vi "Init Sv.vi"   [LabVIEW 2019]
uses:
  TypeDef/SensorCalibrationData_Array.ctl
  TypeDef/SensorCalibrationData.ctl
  TypeDef/CalbrationPoint.ctl
  TypeDef/GUI Alarm customer settings.ctl
  TypeDef/GUI Alarm developer settings.ctl
  TypeDef/GUI Setting Channel.ctl
  TypeDef/Needle Valve Settings.ctl
  modbus engine custom/MB_ENGINE_class/Settings.ctl
  TypeDef/Channel Setting Array.ctl
  modbus engine custom/MB_ENGINE_class/MB_ENGINE.lvclass
types:
  T1 = typedef "Needle Valve Settings.ctl" = cluster{"average size":i32, "open force":u16, "close force":u16, "open settings":T2, "close settings":T2}
  T2 = typedef "MB_ENGINE.lvclass/Settings.ctl" = cluster{"ACC Steps Per Sec^2":u16, "DEC Steps Per Sec^2":u16, "Min Velosity Step Per Sec":u16, "Max Velosity Step Per Sec":u16, "MicroStep":u16}
  T3 = typedef "GUI Setting Channel.ctl" = cluster{"Name":string, "SensorID":u32}
  T4 = typedef "GUI Alarm developer settings.ctl" = cluster{"HIHI AI2":dbl, "HI AI2":dbl, "HIHI AI0":dbl, "HI AI0":dbl, "LOLO AI0":dbl, "LO AI0":dbl, "ENG2 OFF TIMEOUT":dbl, "ENG2 ON TIMEOUT":dbl, "HIHI AI3":dbl, "HI AI3":dbl, "HIHI AI1":dbl, "HI AI1":dbl, "LOLO AI1":dbl, "LO AI1":dbl, "ENG1 OFF TIMEOUT":dbl, "ENG1 ON TIMEOUT":dbl, "ENG0 OFF TIMEOUT":dbl, "ENG0 ON TIMEOUT":dbl, "LOLO AI8":dbl, "LO AI8":dbl, "LOLO AI9":dbl, "LO AI9":dbl, "LOLO AI5":dbl, "LO AI5":dbl, "Out Of Range HI":dbl, "Out Of Range LO":dbl}
  T5 = typedef "GUI Alarm customer settings.ctl" = cluster{"HIHI AI2":dbl, "HI AI2":dbl, "HIHI AI3":dbl, "HI AI3":dbl, "ENG0 OFF TIMEOUT":dbl, "ENG0 ON TIMEOUT":dbl, "HIHI AI7":dbl, "HI AI7":dbl, "HIHI AI6":dbl, "HI AI6":dbl, "HIHI AI5":dbl, "HI AI5":dbl}
  T6 = typedef "SensorCalibrationData_Array.ctl" = cluster{"SENSORS_ARR":T7[]}
  T7 = typedef "SensorCalibrationData.ctl" = cluster{"Name":string, "ID":u32, "Slope":dbl, "Intercept":dbl, "Calibration":T8[]}
  T8 = typedef "CalbrationPoint.ctl" = cluster{"RAW":dbl, "SCL":dbl}
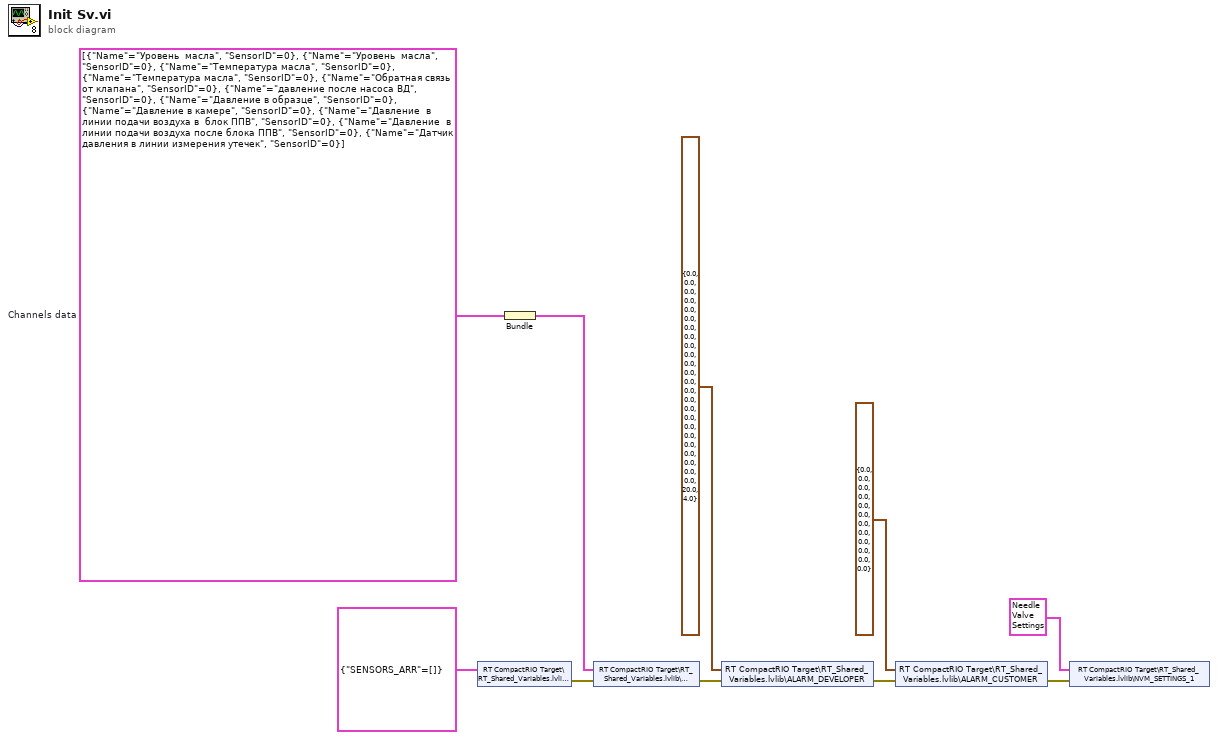
[diagram p0: block diagram]
diagram:
  w4 = T3[] [{"Name"="Уровень  масла", "SensorID"=0}, {"Name"="Уровень  масла", "SensorID"=0}, {"Name"="Температура масла", "SensorID"=0}, {"Name"="Температура масла", "SensorID"=0}, {"Name"="Обратная связь от клапана", "SensorID"=0}, {"Name"="давление после насоса ВД", "SensorID"=0}, {"Name"="Давление в образце", "SensorID"=0}, {"Name"="Давление в камере", "SensorID"=0}, {"Name"="Давление  в  линии подачи воздуха в  блок ППВ", "SensorID"=0}, {"Name"="Давление  в  линии подачи воздуха после блока ППВ", "SensorID"=0}, {"Name"="Датчик давления в линии измерения утечек", "SensorID"=0}]  # Channels data
  n1 = shared-variable "RT CompactRIO Target\\RT_Shared_Variables.lvlib\\SENSORS"(T6 {"SENSORS_ARR"=[]} ("SENSORS")) -> (error out=w9:errorcluster)  [unwired: 1 in]
  n2 = Bundle("Channels data"=w4) -> (w3:cluster{"Channels data":T3[]})  [unwired: 1 in]
  n3 = shared-variable "RT CompactRIO Target\\RT_Shared_Variables.lvlib\\CHANNELS"(w3, error in=w9) -> (error out=w6:errorcluster)
  n4 = shared-variable "RT CompactRIO Target\\RT_Shared_Variables.lvlib\\ALARM_DEVELOPER"(T4 {"HIHI AI2"=0.0, "HI AI2"=0.0, "HIHI AI0"=0.0, "HI AI0"=0.0, "LOLO AI0"=0.0, "LO AI0"=0.0, "ENG2 OFF TIMEOUT"=0.0, "ENG2 ON TIMEOUT"=0.0, "HIHI AI3"=0.0, "HI AI3"=0.0, "HIHI AI1"=0.0, "HI AI1"=0.0, "LOLO AI1"=0.0, "LO AI1"=0.0, "ENG1 OFF TIMEOUT"=0.0, "ENG1 ON TIMEOUT"=0.0, "ENG0 OFF TIMEOUT"=0.0, "ENG0 ON TIMEOUT"=0.0, "LOLO AI8"=0.0, "LO AI8"=0.0, "LOLO AI9"=0.0, "LO AI9"=0.0, "LOLO AI5"=0.0, "LO AI5"=0.0, "Out Of Range HI"=20.0, "Out Of Range LO"=4.0} ("ALARM_DEVELOPER"), error in=w6) -> (error out=w5:errorcluster)
  n5 = shared-variable "RT CompactRIO Target\\RT_Shared_Variables.lvlib\\ALARM_CUSTOMER"(T5 {"HIHI AI2"=0.0, "HI AI2"=0.0, "HIHI AI3"=0.0, "HI AI3"=0.0, "ENG0 OFF TIMEOUT"=0.0, "ENG0 ON TIMEOUT"=0.0, "HIHI AI7"=0.0, "HI AI7"=0.0, "HIHI AI6"=0.0, "HI AI6"=0.0, "HIHI AI5"=0.0, "HI AI5"=0.0} ("ALARM_CUSTOMER"), error in=w5) -> (error out=w1:errorcluster)
  n6 = shared-variable "RT CompactRIO Target\\RT_Shared_Variables.lvlib\\NVM_SETTINGS_1"(T1 {"average size"=0, "open force"=12, "close force"=12, "open settings"={"ACC Steps Per Sec^2"=50, "DEC Steps Per Sec^2"=50, "Min Velosity Step Per Sec"=100, "Max Velosity Step Per Sec"=200, "MicroStep"=16}, "close settings"={"ACC Steps Per Sec^2"=0, "DEC Steps Per Sec^2"=0, "Min Velosity Step Per Sec"=0, "Max Velosity Step Per Sec"=0, "MicroStep"=0}} ("NVM_SETTINGS_1"), error in=w1) -> ()  [unwired: 1 out]
